vi "create array of lines 2.vi"(10 "object":T1 {"direction" step=0.1}) -> (2 "lines[]":cluster{"y":i32, "x start":i32, "x end":i32}[](array[cluster]))   [LabVIEW 2009]
uses:
  object.ctl
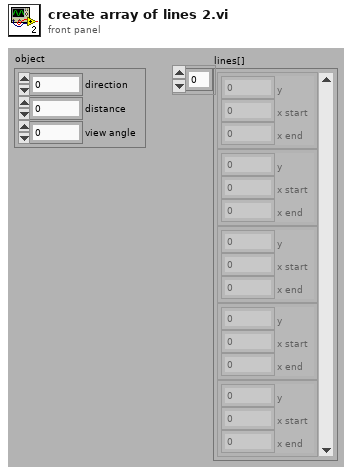
[diagram p1: front panel]
types:
  T1 = typedef "object.ctl" = cluster{"direction":dbl, "distance":u32, "view angle":dbl}
  T2 = typedef "direction info.ctl" = cluster{"above x axis":bool, "left edge":bool}
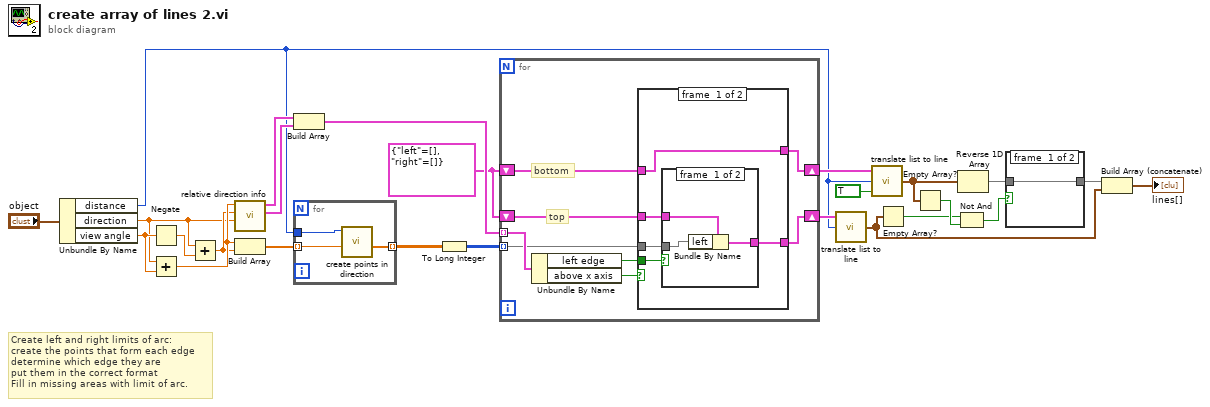
[diagram p0: block diagram]
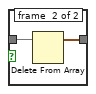
[diagram p2: hidden frame]
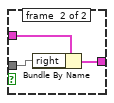
[diagram p3: hidden frame]
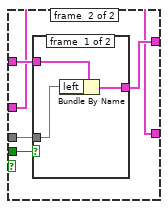
[diagram p4: hidden frame]
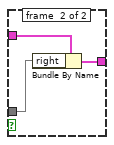
[diagram p5: hidden frame]
diagram:
  w14 = cluster{"left":i32[], "right":i32[]} {"left"=[], "right"=[]}
  # "Create left and right limits of arc:\ncreate the points that form each edge\ndetermine which edge they are\nput them in the correct format\nFill in missing areas with limit of arc."
  n1 = Unbundle By Name("object") -> ("distance"=w9:u32, "direction"=w19:dbl, "view angle"=w23:dbl)
  n2 = Negate(x=w23) -> (-x=w24:dbl)
  n3 = Add(x=w19, y=w23) -> (x+y=w21:dbl)
  n4 = Add(x=w19, y=w24) -> (x+y=w20:dbl)
  n5 = call "relative direction info.vi"("central direction"=w19, "direction 2"=w20, "direction 1"=w21) -> ("direction 2 info"=w17:T2, "direction 1 info"=w18:T2)  [unwired: 7 in]
  n6 = Build Array(w21, w20) -> (w22:dbl[])
  n7 = Build Array(w18, w17) -> (w15:T2[])
  n8 = for {
    tunnel: w22 -> [w28] mode=indexing
    tunnel: w9 -> [w27]
    tunnel: [w26] -> w16 mode=indexing
    n9 = call "create points in direction.vi"("angle"=w28, "distance"=w27) -> ("x values"=w26:dbl[])  [unwired: 8 in, 1 out]
  }
  n10 = To Long Integer(number=w16) -> (32bit integer=w12:i32[][])
  n11 = for {
    tunnel: w12 -> [w35] mode=indexing
    tunnel: w15 -> [w36] mode=indexing
    shift-right: [w31] -> w13
    shift-left: w14 -> [w33]
    shift-right: [w30] -> w11
    shift-left: w14 -> [w32]
    # "bottom"
    # "top"
    n12 = Unbundle By Name(w36) -> ("left edge"=w34:bool, "above x axis"=w29:bool)
    n13 = case shown="False" w29 {
      tunnel: w35 -> [w41 w52]
      tunnel: w34 -> [w40 w51]
      tunnel: w33 -> [w39 w48]
      tunnel: w32 -> [w37 w50]
      tunnel: [w38 w48] -> w31
      tunnel: [w37 w49] -> w30
      frame #0 {
        n14 = case shown="False" w40 {
          tunnel: w41 -> [w43 w46]
          tunnel: w39 -> [w44 w47]
          tunnel: [w42 w45] -> w38
          frame #0 {
            n15 = Bundle By Name(cluster=w44, "left"=w43) -> (w42:cluster{"left":i32[], "right":i32[]})
          }
          frame #1 {
            n16 = Bundle By Name(cluster=w47, "right"=w46) -> (w45:cluster{"left":i32[], "right":i32[]})
          }
        }
      }
      frame #1 {
        n17 = case shown="True" w51 {
          tunnel: w52 -> [w54 w57]
          tunnel: w50 -> [w55 w58]
          tunnel: [w53 w56] -> w49
          frame #0 {
            n18 = Bundle By Name(cluster=w55, "left"=w54) -> (w53:cluster{"left":i32[], "right":i32[]})
          }
          frame #1 {
            n19 = Bundle By Name(cluster=w58, "right"=w57) -> (w56:cluster{"left":i32[], "right":i32[]})
          }
        }
      }
    }
  }
  n20 = call "translate list to line.vi"("distance"=w9, "list"=w13) -> ("Array"=w2:cluster{"y":i32, "x start":i32, "x end":i32}[])  [unwired: 3 in]
  n21 = call "translate list to line.vi"("negate y (false)"=TRUE, "distance"=w9, "list"=w11) -> ("Array"=w7:cluster{"y":i32, "x start":i32, "x end":i32}[])  [unwired: 2 in]
  n22 = Empty Array?(array=w2) -> (empty?=w5:bool)
  n23 = Empty Array?(array=w7) -> (empty?=w6:bool)
  n24 = Not And(1:w6, 2:w5) -> (0:w4:bool)
  n25 = Reverse 1D Array(array=w7) -> (reversed array=w8:cluster{"y":i32, "x start":i32, "x end":i32}[])
  n26 = case shown="False" w4 {
    tunnel: w8 -> [w59 w61]
    tunnel: [w59 w60] -> w3
    frame #0 {
    }
    frame #1 {
      n27 = Delete From Array(array=w61) -> (array with subset deleted=w60:cluster{"y":i32, "x start":i32, "x end":i32}[])  [unwired: 2 in, 1 out]
    }
  }
  n28 = Build Array (concatenate)(w3, w2) -> (→"lines[]":cluster{"y":i32, "x start":i32, "x end":i32}[])
